vi "getDeviceStatus.vi"(8 "error in (no error)":errorcluster, 11 "tcpExampleControler in":refnum<class "tcpExampleControler.lvclass">) -> (0 "error out":errorcluster, 2 "status":T1, 3 "tcpExampleControler out":refnum<class "tcpExampleControler.lvclass">)   [LabVIEW 2016, in "tcpExampleControler.lvclass"]
uses:
  tcpExampleControler.lvclass
  C:/Users/aanania/Documents/common_labview_tcpdevice/tcpDevice/tcpDevice.lvclass
  typedefs/deviceStatus.ctl
  typedefs/statusEnum.ctl
  tcpDevice/tcpDevice.lvclass
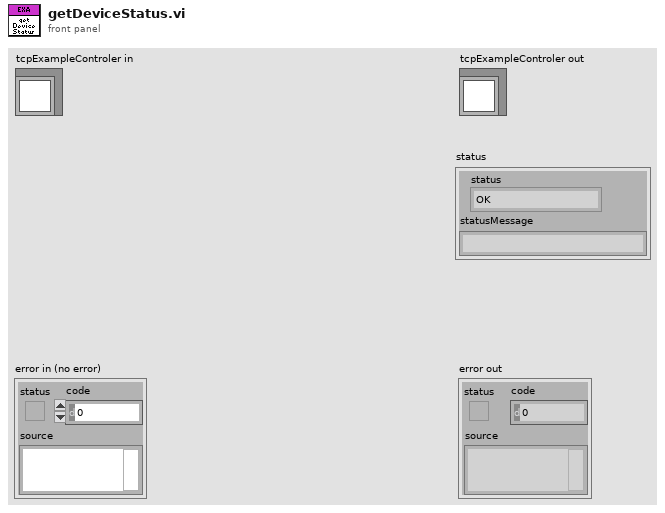
[diagram p1: front panel]
types:
  T1 = typedef "deviceStatus.ctl" = cluster{"status":T2, "statusMessage":string}
  T2 = typedef "statusEnum.ctl" = enum16{"OK", "TIMEOUT", "MSGERROR"}
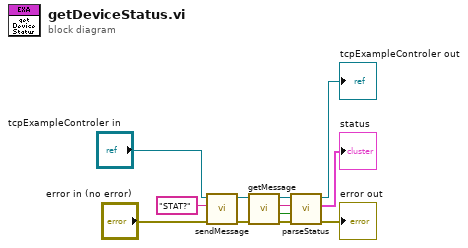
[diagram p0: block diagram]
diagram:
  n1 = call "sendMessage.vi"("error in (no error)"="error in (no error)", "Message"="STAT?", "tcpDevice in"="tcpExampleControler in") -> ("error out"=w11:errorcluster, "tcpDevice out"=w9:refnum<class "tcpExampleControler.lvclass">)  [unwired: 7 in]
  n2 = call "getMessage.vi"("error in (no error)"=w11, "tcpDevice in"=w9) -> ("error out"=w4:errorcluster, "timeout"=w5:bool, "Message"=w6:string, "tcpDevice out"=w7:refnum<class "tcpExampleControler.lvclass">)  [unwired: 6 in]
  n3 = call-dynamic "parseStatus.vi"("error in (no error)"=w4, "timeout"=w5, "Message"=w6, "tcpExampleControler in"=w7) -> ("error out"=→"error out":errorcluster, "status"=→"status":T1, "tcpExampleControler out"=→"tcpExampleControler out":refnum<class "tcpExampleControler.lvclass">)  [unwired: 5 in]
